vi "Actor Core.vi"(8 "error in":errorcluster, 11 "UserInterface in":refnum<class "UserInterface.lvclass">) -> (0 "error out":errorcluster, 3 "Actor out":refnum<class "Actor.lvclass">)   [LabVIEW 2016, in "UserInterface.lvlib" / "UserInterface.lvclass"]
doc: "(<B>Filename</B>: Actor Framework.lvlib:Actor.lvclass:Actor Core.vi)\n\nReceives messages to the actor, reacts to them, and initiates any error handling that may shut the actor down.\n\nDescendant classes may override this VI to append parallel tasks for the actor to complete while it handles messages. Overrides use the Call Parent Method node."
uses:
  UserInterface.lvclass
  C:/Program Files/National Instruments/LabVIEW 2016/vi.lib/ActorFramework/Actor/Actor.lvclass
  <vilib>/ActorFramework/Actor/Actor.lvclass
  UserInterface.lvclass/UserInterface.ctl
  <vilib>/ActorFramework/Actor/Actor.lvclass/Actor.ctl
  <vilib>/ActorFramework/Message Enqueuer/Message Enqueuer.lvclass/Message Enqueuer.ctl
  <vilib>/ActorFramework/Message Enqueuer/Enqueue.vi
  <vilib>/ActorFramework/Stop Msg/Stop Msg.lvclass
  C:/Program Files/National Instruments/LabVIEW 2016/vi.lib/ActorFramework/Message/Message.lvclass
  <vilib>/ActorFramework/Message Priority Queue/Priority Enqueue.vi
panel:
  in  "Table Control":string[][](table)
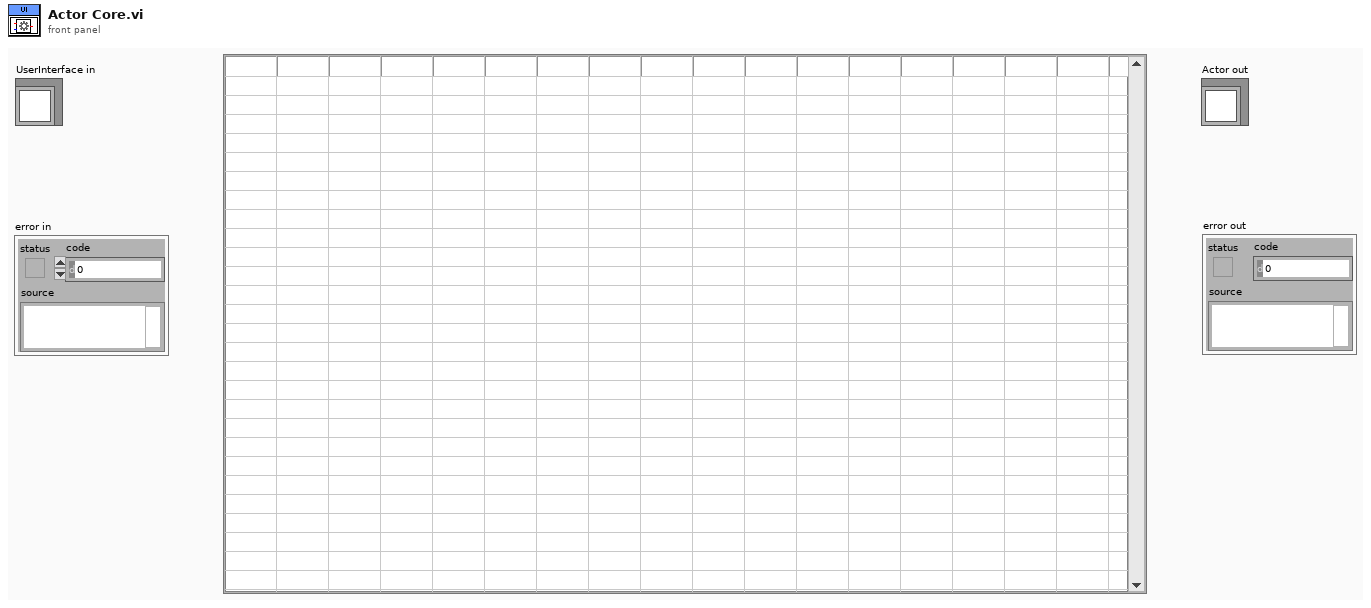
[diagram p1: front panel]
types:
  T1 = typedef "LVPoint32TypeDef.ctl" = cluster{"Horizontal":i32, "Vertical":i32}
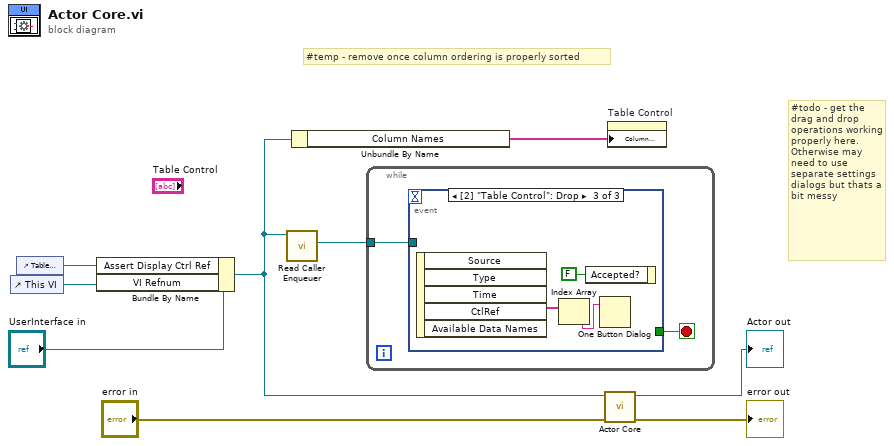
[diagram p0: block diagram]
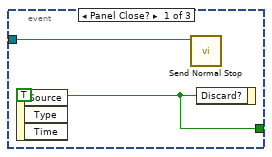
[diagram p2: hidden frame]
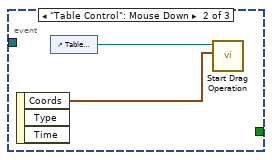
[diagram p3: hidden frame]
diagram:
  # "#todo - get the drag and drop operations working properly here. Otherwise may need to use separate settings dialogs but thats a bit messy"
  # "#temp - remove once column ordering is properly sorted"
  n1 = control-ref of="This VI"() -> (w4:refnum<vi>)
  n2 = control-ref of="Table Control"() -> (w3:refnum<vi>)
  n3 = Bundle By Name(cluster="UserInterface in", "Assert Display Ctrl Ref"=w3, "VI Refnum"=w4) -> (w2:refnum<class "UserInterface.lvclass">)
  n4 = call <vilib>:"Read Caller Enqueuer.vi"("Actor"=w2) -> ("Caller Enqueuer"=w5:refnum<class "Message Enqueuer.lvclass">)  [unwired: 10 in]
  n5 = Unbundle By Name(w2) -> ("Column Names"=w1:string[])
  n6 = while {
    tunnel: w5 -> [w10]
    stop <- w11 stop-if-true
    n7 = event shown="[2] \"Table Control\": Drop" {
      selector: _ -> [_ _ _]
      dyn-events: _ -> [_ _ _]
      timeout: _ -> [_ _ _]
      tunnel: [w13 _ _] -> w11
      tunnel: w10 -> [w12 _ _]
      event Panel Close? {
        w13 = TRUE ("Discard?")
        n8 = event-data() -> ()  [unwired: 1 in, 3 out]
        n9 = call <vilib>:"Send Normal Stop.vi"("Message Enqueuer"=w12) -> ()  [unwired: 10 in, 1 out]
        n10 = event-data("Discard?"=w13) -> ()  [unwired: 1 in, 1 out]
      }
      event "Table Control": Mouse Down {
        n11 = event-data() -> ("Coords"=w15:T1)  [unwired: 1 in, 2 out]
        n12 = control-ref of="Table Control"() -> (w14:refnum<vi>)
        n13 = call "Start Drag Operation.vi"("Coords"=w15, "Table in"=w14) -> ()  [unwired: 9 in, 1 out]
      }
      event "Table Control": Drop {
        n14 = event-data() -> ("Available Data Names"=w17:string[])  [unwired: 1 in, 4 out]
        n15 = Index Array(array=w17) -> (element=w16:string)  [unwired: 1 in]
        n16 = event-data("Accepted?"=FALSE) -> ()  [unwired: 1 in, 1 out]
        n17 = One Button Dialog(message=w16) -> ()  [unwired: 1 in, 1 out]
      }
    }
  }
  n18 = call-parent "Actor Core.vi"("error in"="error in", "Actor in"=w2) -> ("error out"=→"error out":errorcluster, "Actor out"=→"Actor out":refnum<class "Actor.lvclass">)  [unwired: 8 in]
  n19 = property on="Table Control" class="Tbl (strict)"("Column Headers[]"=w1) -> ()  [unwired: 2 in, 2 out]
